vi "Transmit.vi"(8 "error in (no error)":errorcluster, 10 "Transfer Group in":refnum<class "Transfer Group.lvclass">, 11 "GE Reflective Memory Transceiver in":refnum<class "GE Reflective Memory Transceiver.lvclass">) -> (0 "error out":errorcluster, 2 "Transfer Group out":refnum<class "Transfer Group.lvclass">, 3 "GE Reflective Memory Transceiver out":refnum<class "GE Reflective Memory Transceiver.lvclass">)   [LabVIEW 2017, in "GE Reflective Memory.lvlib" / "GE Reflective Memory Transceiver.lvclass"]
uses:
  GE Reflective Memory Transceiver.lvclass
  Builds/Data Sharing Framework/Current/Core/DSF Core.lvlibp/Classes/Transfer Group/Transfer Group.lvclass
  GE Reflective Memory Transceiver.lvclass/GE Reflective Memory Transceiver.ctl
  <vilib>/NI/GE Reflective Memory Driver/GE 5565PIORC.lvclass/GE 5565PIORC.ctl
  <vilib>/NI/GE Reflective Memory Driver/Methods/GE 5565PIORC.DMA.Configure.vi
  <vilib>/NI/GE Reflective Memory Driver/Methods/GE 5565PIORC.PXI Interrupts.Discard Events.vi
  <vilib>/NI/GE Reflective Memory Driver/Methods/GE 5565PIORC.DMA.Start.vi
  <vilib>/NI/GE Reflective Memory Driver/Methods/GE 5565PIORC.DMA.Wait for Done.vi
  <vilib>/NI/GE Reflective Memory Driver/Properties/Registers/GE 5565PIORC.Registers.DMADPR0.Direction of Transfer.Set.vi
  <vilib>/NI/GE Reflective Memory Driver/Properties/Registers/GE 5565PIORC.Registers.DMASIZ0.DMA Transfer Size.Set.vi
  <vilib>/NI/GE Reflective Memory Driver/Methods/GE 5565PIORC.DMA.Size.vi
  <vilib>/NI/GE Reflective Memory Driver/Properties/Registers/GE 5565PIORC.Registers.DMALADR0.Local Address Register.Set.vi
  <vilib>/NI/GE Reflective Memory Driver/Properties/Registers/GE 5565PIORC.Registers.DMAMODE0.Scatter-Gather Mode.Set.vi
  <vilib>/NI/GE Reflective Memory Driver/Properties/Registers/GE 5565PIORC.Registers.DMAPADR0.PCI Address Register.Set.vi
  <vilib>/NI/GE Reflective Memory Driver/Methods/GE 5565PIORC.DMA.Scatter-Gather.Link Block Descriptors.vi
  <vilib>/NI/GE Reflective Memory Driver/Methods/GE 5565PIORC.DMA.Scatter-Gather.Commit Linked Block Descriptors.vi
  <vilib>/NI/GE Reflective Memory Driver/Properties/Registers/GE 5565PIORC.Registers.DMADPR0.Channel 0 First Descriptor Address.Set.vi
  <vilib>/NI/GE Reflective Memory Driver/Methods/GE 5565PIORC.DMA.Get Transfer Components.vi
  <vilib>/NI/GE Reflective Memory Driver/Methods/GE 5565PIORC.DMA.Get Transfer Components (Scatter-Gather).vi
  <vilib>/Utility/error.llb/Clear Errors.vi
  <vilib>/NI/GE Reflective Memory Driver/Properties/Registers/GE 5565PIORC.Registers.DMACSR0.Channel 0 Start.Set.vi
  <vilib>/NI/GE Reflective Memory Driver/Properties/Registers/GE 5565PIORC.Registers.DMACSR0.Channel 0 Clear Interrupt.Set.vi
  <vilib>/NI/GE Reflective Memory Driver/Methods/GE 5565PIORC.DMA.Poll for Done Signal.vi
  <vilib>/NI/GE Reflective Memory Driver/Methods/GE 5565PIORC.PXI Interrupts.Wait for Event.vi
  <vilib>/NI/GE Reflective Memory Driver/Properties/Registers/GE 5565PIORC.Registers.Local Configuration.Read.vi
  <vilib>/NI/GE Reflective Memory Driver/Properties/Registers/GE 5565PIORC.Registers.Local Configuration.Read (U32).vi
  <vilib>/NI/GE Reflective Memory Driver/Properties/Registers/GE 5565PIORC.Registers.Local Configuration.Write.vi
  <vilib>/NI/GE Reflective Memory Driver/Properties/Registers/GE 5565PIORC.Registers.Local Configuration.Write (U32).vi
  <vilib>/NI/GE Reflective Memory Driver/Methods/GE 5565PIORC.Bit Manipulation.Set Bit.vi
  <vilib>/NI/GE Reflective Memory Driver/Methods/GE 5565PIORC.Bit Manipulation.Set Bit (U32).vi
  <vilib>/NI/GE Reflective Memory Driver/Methods/GE 5565PIORC.DMA.Scatter-Gather.Set Descriptor Params.vi
  <vilib>/NI/GE Reflective Memory Driver/Properties/Registers/GE 5565PIORC.Registers.Local Configuration.Read (U8).vi
  <vilib>/NI/GE Reflective Memory Driver/Properties/Registers/GE 5565PIORC.Registers.Local Configuration.Write (U8).vi
  <vilib>/NI/GE Reflective Memory Driver/Methods/GE 5565PIORC.Bit Manipulation.Set Bit (U8).vi
  <vilib>/NI/GE Reflective Memory Driver/Methods/GE 5565PIORC.DMA.Is Done.vi
  <vilib>/NI/GE Reflective Memory Driver/Methods/GE 5565PIORC.Registers.Read.vi
  <vilib>/NI/GE Reflective Memory Driver/Methods/GE 5565PIORC.Registers.Read (U32).vi
  <vilib>/NI/GE Reflective Memory Driver/Methods/GE 5565PIORC.Registers.Write.vi
  <vilib>/NI/GE Reflective Memory Driver/Methods/GE 5565PIORC.Registers.Write (U32).vi
  <vilib>/NI/GE Reflective Memory Driver/Methods/GE 5565PIORC.Registers.Read (U8).vi
  <vilib>/NI/GE Reflective Memory Driver/Methods/GE 5565PIORC.Registers.Write (U8).vi
  <vilib>/NI/GE Reflective Memory Driver/Properties/Registers/GE 5565PIORC.Registers.DMACSR0.Channel 0 Inactive.Get.vi
  <vilib>/NI/GE Reflective Memory Driver/Methods/GE 5565PIORC.Bit Manipulation.Get Bit.vi
  <vilib>/NI/GE Reflective Memory Driver/Methods/GE 5565PIORC.Bit Manipulation.Get Bit (U8).vi
  <vilib>/NI/GE Reflective Memory Driver/GE 5565PIORC.lvclass
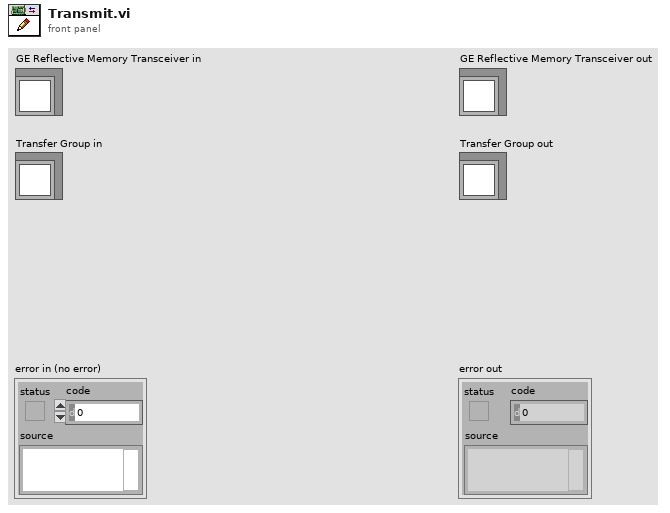
[diagram p1: front panel]
types:
  T1 = typedef "GE Reflective Memory.lvlib/GE Reflective Memory Transceiver.lvclass/Transfer Group Parameters.ctl" = cluster{"DMA Transfer Specs":T2[]}
  T2 = typedef "GE 5565PIORC.lvclass/GE 5565PIORC.Typedef.DMA Transfer Spec.ctl" = cluster{"RFM offset":u32, "Block Descriptors":T3[]}
  T3 = typedef "GE 5565PIORC.lvclass/GE 5565PIORC.Typedef.DMA Block Descriptor.ctl" = cluster{"descriptor ptr (VISA)":u32, "descriptor ptr (RFM)":u32, "descriptor size":u32, "descriptor params":T4}
  T4 = typedef "GE 5565PIORC.lvclass/GE 5565PIORC.Typedef.DMA Block Descriptor Params.ctl" = cluster{"data ptr (lower)":u32, "data ptr (upper)":u32, "data size":u32, "next descriptor ptr":u32}
  T5 = typedef "GE 5565PIORC.lvclass/GE 5565PIORC.Typedef.DMA Wait Mode.ctl" = enum16{"Polling", "Interrupt"}
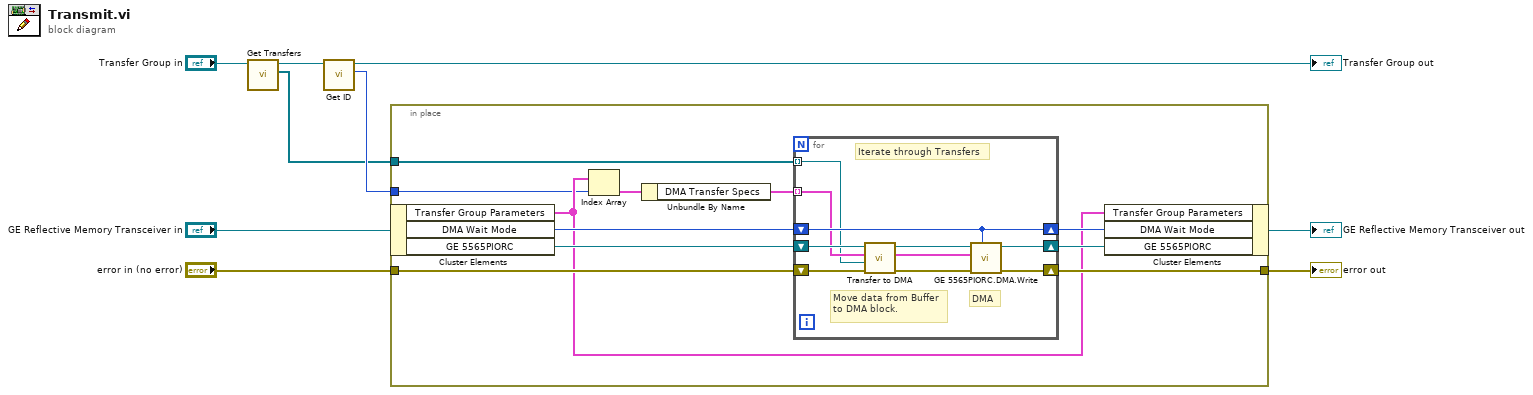
[diagram p0: block diagram]
diagram:
  n1 = call "Get Transfers.vi"("Transfer Group in"="Transfer Group in") -> ("Transfers"=w5:refnum<class "Transfer.lvclass">[], "Transfer Group out"=w4:refnum<class "Transfer Group.lvclass">)  [unwired: 9 in]
  n2 = call "Get ID.vi"("Transfer Group in"=w4) -> ("id"=w6:i32, "Transfer Group out"=→"Transfer Group out":refnum<class "Transfer Group.lvclass">)  [unwired: 9 in]
  n3 = in-place {
    in-place-border: "error in (no error)" -> [w19]
    in-place-border: [w18] -> w8
    in-place-border: w6 -> [w13]
    in-place-border: w5 -> [w12]
    n4 = in-place-cluster #1("GE Reflective Memory Transceiver in") -> ("Transfer Group Parameters"=w14:T1[], "DMA Wait Mode"=w16:T5, "GE 5565PIORC"=w20:refnum<class "GE 5565PIORC.lvclass">)
    n5 = Index Array(array=w14, index=w13) -> (element=w11:T1)
    n6 = Unbundle By Name(w11) -> ("DMA Transfer Specs"=w10:T2[])
    n7 = for {
      shift-right: [w29] -> w17
      shift-left: w20 -> [w27]
      shift-right: [w30] -> w18
      shift-left: w19 -> [w26]
      shift-right: [w28] -> w15
      shift-left: w16 -> [w28]
      tunnel: w10 -> [w25] mode=indexing
      tunnel: w12 -> [w21] mode=indexing
      # "Iterate through Transfers"
      # "DMA"
      # "Move data from Buffer to DMA block."
      n8 = call "Transfer to DMA.vi"("error in (no error)"=w26, "Transfer in"=w21, "DMA Transfer Spec in"=w25, "GE 5565PIORC in"=w27) -> ("error out"=w22:errorcluster, "DMA Transfer Spec out"=w24:T2, "GE 5565PIORC out"=w23:refnum<class "GE 5565PIORC.lvclass">)  [unwired: 4 in, 1 out]
      n9 = call <vilib>:"GE 5565PIORC.DMA.Write.vi"("wait mode (polling)"=w28, "error in (no error)"=w22, "DMA Transfer Spec"=w24, "GE 5565PIORC in"=w23) -> ("error out"=w30:errorcluster, "GE 5565PIORC out"=w29:refnum<class "GE 5565PIORC.lvclass">)  [unwired: 4 in, 2 out]
    }
    n10 = in-place-cluster #1("Transfer Group Parameters"=w14, "DMA Wait Mode"=w15, "GE 5565PIORC"=w17) -> (→"GE Reflective Memory Transceiver out":refnum<class "GE Reflective Memory Transceiver.lvclass">)
  }
  "error out" <- w8
